vi "Obtain SEQ.vi"(8 "error in":errorcluster, 11 "Module ID":i32) -> (0 "error out":errorcluster, 2 "Created New?":bool, 3 "Local Instance Event SEQ":refnum<queue>)   [LabVIEW 2019, in "Inversor.lvlib" / "Local Instance Events SEQ.lvlib"]
doc: "_____\nCreated using DQMH Framework: Event Scripter 7.1.0.1503."
uses:
  Local Instance Events SEQ.lvlib
  Local Instance Request Events--cluster.ctl
  Request Privado Local Argument--cluster.ctl
  Inversor.lvlib
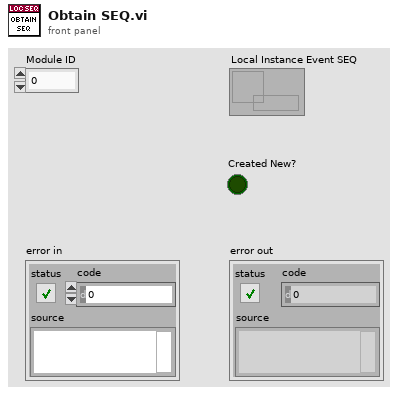
[diagram p1: front panel]
types:
  T1 = typedef "Inversor.lvlib/Local Instance Request Events--cluster.ctl" = cluster{"Request Privado Local":refnum<user-event>}
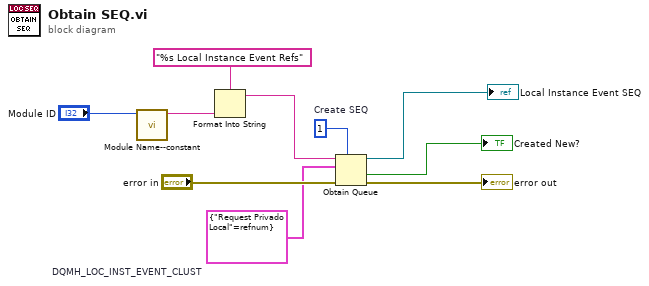
[diagram p0: block diagram]
diagram:
  w4 = T1 {"Request Privado Local"=refnum}  # DQMH_LOC_INST_EVENT_CLUST
  w7 = 1  # Create SEQ
  n1 = call "Module Name--constant.vi"("Module ID"="Module ID") -> ("Module Name"=w1:string)  [unwired: 10 in]
  n2 = Format Into String(format string="%s Local Instance Event Refs", w1) -> (resulting string=w6:string)  [unwired: 2 in, 1 out]
  n3 = Obtain Queue(max queue size (-1, unlimited)=w7, name (unnamed)=w6, element data type=w4, error in (no error)="error in") -> (queue out=→"Local Instance Event SEQ":refnum<queue>, created new?=→"Created New?":bool, error out=→"error out":errorcluster)  [unwired: 1 in]
